vi "Reset.vi"(8 "Error In":errorcluster, 11 "Timer Handle":T1) -> (0 "Error Out":errorcluster, 3 "Timer Handle":T1)   [LabVIEW 2021, in "Timer-API.lvlib" / "Timer Session.lvclass"]
doc: "Resets the timer.\n\nYou can specify the input as timer name or timer reference. Using reference executes faster."
uses:
  Timer Session.lvclass
  Timer Session.lvclass/Timer Session.ctl
  Typedefs/Session Handle.ctl
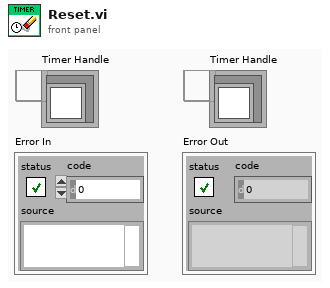
[diagram p1: front panel]
types:
  T1 = typedef "Timer-API.lvlib/Timer Session.lvclass/Session Handle.ctl" = refnum<data-value>
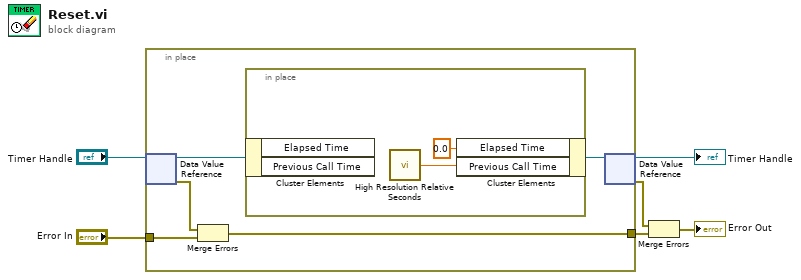
[diagram p0: block diagram]
diagram:
  n1 = in-place {
    in-place-border: "Error In" -> [w8]
    in-place-border: [w7] -> w3
    n2 = in-place-dvr #1("Timer Handle") -> (w11:refnum<class "Timer Session.lvclass">, w9:errorcluster)
    n3 = Merge Errors(w9, w8) -> (w7:errorcluster)
    n4 = in-place {
      n5 = in-place-cluster #2(w11) -> ()  [unwired: 2 out]
      n6 = call <vilib>:"High Resolution Relative Seconds.vi"() -> ("relative seconds"=w12:dbl)
      n7 = in-place-cluster #2("Elapsed Time"=0.0 ("Elapsed Time (s)"), "Previous Call Time"=w12) -> (w10:refnum<class "Timer Session.lvclass">)
    }
    n8 = in-place-dvr #1(w10) -> (→"Timer Handle":T1, w2:errorcluster)
  }
  n9 = Merge Errors(w2, w3) -> (→"Error Out":errorcluster)
